vi "Rayleigh PDF.vi"(10 "b":dbl=1.0, 11 "x":dbl=1.0) -> (0 "error":i32, 3 "pdf(x)":dbl=0.6065306597126334)   [LabVIEW 2020, in "NI_Gmath.lvlib"]
doc: "Computes the continuous probability density function (PDF) of various distributions. You must manually select the polymorphic instance to use."
uses:
  <vilib>/gmath/NI_Gmath.lvlib
  <vilib>/gmath/statdist.llb/st_error_code.ctl
panel:
  # "Rayleigh PDF"
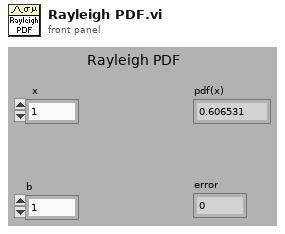
[diagram p1: front panel]
types:
  T1 = typedef "NI_Gmath.lvlib/st_error_code.ctl" = i32
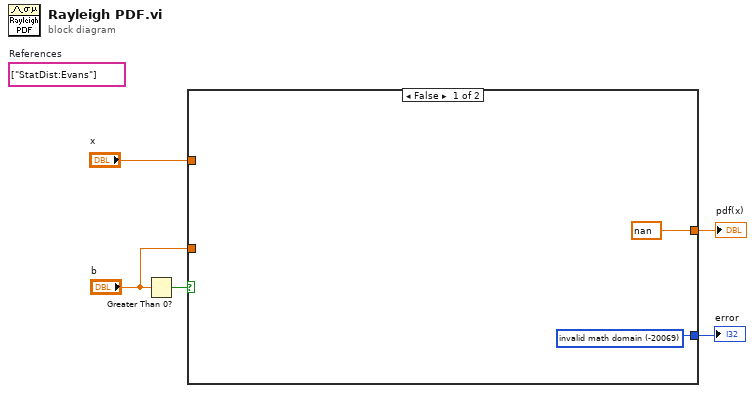
[diagram p0: block diagram]
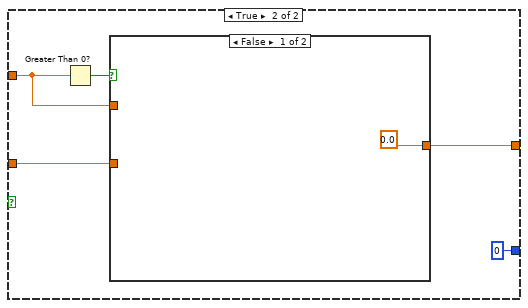
[diagram p2: hidden frame]
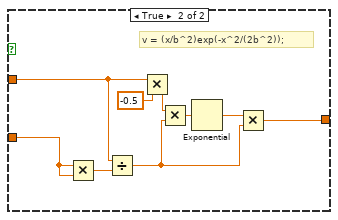
[diagram p3: hidden frame]
diagram:
  (unwired) string[] ["StatDist:Evans"]  # References
  n1 = Greater Than 0?(x="b") -> (x > 0?=w2:bool)
  n2 = case shown="False" w2 {
    tunnel: "b" -> [_ w10]
    tunnel: [w6 0 ("invalid math domain")] -> w5
    tunnel: [nan w11] -> w4
    tunnel: "x" -> [_ w8]
    frame False {
      w6 = T1 -20069 items=["invalid math domain"=-20069, "Fourier interpolation size m >= n"=-20070, "empty array"=-20003] ("stat interp error code")
    }
    frame True {
      n3 = Greater Than 0?(x=w8) -> (x > 0?=w9:bool)
      n4 = case shown="False" w9 {
        tunnel: [0.0 w14] -> w11
        tunnel: w8 -> [_ w20]
        tunnel: w10 -> [_ w22]
        frame False {
        }
        frame True {
          # "v = (x/b^2)exp(-x^2/(2b^2));"
          n5 = Multiply(x=w22, y=w22) -> (x*y=w21:dbl)
          n6 = Divide(x=w20, y=w21) -> (x/y=w16:dbl)
          n7 = Multiply(x=w20, y=-0.5) -> (x*y=w18:dbl)
          n8 = Multiply(x=w18, y=w16) -> (x*y=w17:dbl)
          n9 = Exponential(1:w17) -> (0:w15:dbl)
          n10 = Multiply(x=w15, y=w16) -> (x*y=w14:dbl)
        }
      }
    }
  }
  "pdf(x)" <- w4
  "error" <- w5
